vi "DecodeUInt16.vi"(1 "Data In":u8[](array[numeric])) -> (0 "Data Out":u16[](array[numeric]))   [LabVIEW 2014, in "navX-MXP IMU.lvlib"]
uses:
  navX-MXP IMU.lvlib
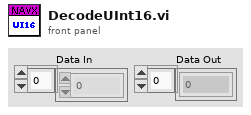
[diagram p1: front panel]
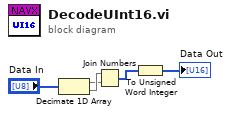
[diagram p0: block diagram]
diagram:
  n1 = Decimate 1D Array("Data In") -> (w3:u8[], w4:u8[])
  n2 = Join Numbers(hi=w4, lo=w3) -> ((hi.lo)=w2:u16[])
  n3 = To Unsigned Word Integer(number=w2) -> (unsigned 16bit integer=→"Data Out":u16[])
